vi "WPI_AccelerometerOpen.vi"   [LabVIEW 2017]
doc: "Opens a reference to the accelerometer you specify. You must open a reference before using any other VIs on this palette."
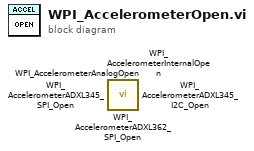
[diagram p0: block diagram]
diagram:
  n1 = call <vilib>:"WPI_AccelerometerADXL362_SPI_Open.vi"() -> ()  [unwired: 10 in, 2 out]
  n2 = call <vilib>:"WPI_AccelerometerInternalOpen.vi"() -> ()  [unwired: 10 in, 2 out]
  n3 = call <vilib>:"WPI_AccelerometerADXL345_SPI_Open.vi"() -> ()  [unwired: 10 in, 2 out]
  n4 = call <vilib>:"WPI_AccelerometerADXL345_I2C_Open.vi"() -> ()  [unwired: 10 in, 2 out]
  n5 = call <vilib>:"WPI_AccelerometerAnalogOpen.vi"() -> ()  [unwired: 10 in, 2 out]
